vi "Begin.vi"(8 "error in":errorcluster) -> (0 "error out":errorcluster)   [LabVIEW 2017]
doc: "Called before other user functions, this VI is expected to open initial I/O refnums, load in file data, and do all program initialization. Notice that the <B>error out</B> terminal is simply used for data flow. Wiring it to other structures or subVIs ensures that this VI runs first."
uses:
  <vilib>/Rock Robotics/WPI/DriverStation/WPI_DriverStationRobotMode2.ctl
  <vilib>/Rock Robotics/WPI/Joystick/WPI_JoystickDeviceEnum.ctl
  <vilib>/Rock Robotics/WPI/Solenoid/WPI_SolenoidChannel.ctl
  <vilib>/Rock Robotics/SystemInterfaces/DIO/FPGA_DIOChannel.ctl
  <vilib>/Rock Robotics/SystemInterfaces/AI/FPGA_AIChannel.ctl
  Desktop/2018 FINAL/E/2018 FINAL/C/Users/admin/Documents/LabVIEW Data/2018 FINAL CODE/Robot Global Data.vi
  <vilib>/Rock Robotics/WPI/Solenoid/WPI_SolenoidOpenDouble.vi
  <vilib>/Rock Robotics/WPI/RobotDrive/WPI_RobotDriveOpen2MotorWithTalonSRX.vi
  <vilib>/Rock Robotics/WPI/ThirdParty/Phoenix-LabVIEW/Pigeon IMU/CTRE_PigeonIMU_Open_TalonSRX.vi
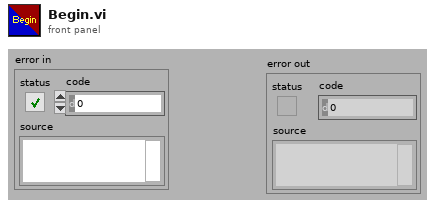
[diagram p1: front panel]
types:
  T1 = typedef "FPGA_AIChannel.ctl" = enum8{"AI 0", "AI 1", "AI 2", "AI 3", "AI MXP 0", "AI MXP 1", "AI MXP 2", "AI MXP 3", "Invalid"}
  T2 = typedef "FPGA_DIOChannel.ctl" = enum8{"DIO 0", "DIO 1", "DIO 2", "DIO 3", "DIO 4", "DIO 5", "DIO 6", "DIO 7", "DIO 8", "DIO 9", "DIO MXP 0", "DIO MXP 1", "DIO MXP 2", "DIO MXP 3", "DIO MXP 4", "DIO MXP 5", "DIO MXP 6", "DIO MXP 7", "DIO MXP 8", "DIO MXP 9", "DIO MXP 10", "DIO MXP 11", "DIO MXP 12", "DIO MXP 13", "DIO MXP 14", "DIO MXP 15", "SPI Port CS1", "SPI Port CS2", "SPI Port CS3", "SPI Port MISO", "SPI Port MOSI", "Invalid"}
  T3 = typedef "WPI_JoystickDeviceEnum.ctl" = enum16{"USB 0", "USB 1", "USB 2", "USB 3", "USB 4", "USB 5"}
  T4 = typedef "WPI_SolenoidChannel.ctl" = enum8{"Solenoid 0", "Solenoid 1", "Solenoid 2", "Solenoid 3", "Solenoid 4", "Solenoid 5", "Solenoid 6", "Solenoid 7", "Invalid"}
  T5 = typedef "WPI_DriverStationRobotMode2.ctl" = enum16{"Autonomous Disabled", "Autonomous Enabled", "Teleop Disabled", "Teleop Enabled", "Disconnected", "Finish", "Test Disabled", "Test Enabled", "Emergency Stopped"}
  T6 = typedef "WPI_MotorControlDeviceRef.ctl" = cluster{"DeviceStatus":errorcluster, "Type":T7, "PWM":cluster{"PWM Channel":T8, "DeadBand":T9}, "CAN":cluster{"Device Number":u8, "SetOutput VI Ref":variant, "GetOutput VI Ref":variant, "Enable VI Ref":variant, "Disable VI Ref":variant, "Data":variant}, "Invert":bool, "DIO PWM":cluster{"PWM \"Enable\" Channel":T8, "DIOChannel":T2, "PWM Rate":dbl}}
  T7 = typedef "WPI_MotorControlType.ctl" = enum16{"PWM", "CAN", "DIO PWM"}
  T8 = typedef "FPGA_DIOPWMChannel.ctl" = enum8{"PWM 0", "PWM 1", "PWM 2", "PWM 3", "PWM 4", "PWM 5", "PWM 6", "PWM 7", "PWM 8", "PWM 9", "PWM MXP 0", "PWM MXP 1", "PWM MXP 2", "PWM MXP 3", "PWM MXP 4", "PWM MXP 5", "PWM MXP 6", "PWM MXP 7", "PWM MXP 8", "PWM MXP 9", "Invalid"}
  T9 = typedef "WPI_PWMDeadband.ctl" = cluster{"Name":string, "maxPositivePwm":i32, "minPositivePwm":i32, "centerPwm":i32, "maxNegativePwm":i32, "minNegativePwm":i32, "angularRange":u16}
  T10 = typedef "WPI_JoystickDevRef.ctl" = cluster{"Device":T3}
  T11 = typedef "WPI_RobotDriveDevRef.ctl" = cluster{"DevStatus":errorcluster, "Motors[]":T6[], "Square Inputs":bool, "Max Output":dbl}
  T12 = typedef "WPI_SolenoidDevRef.ctl" = cluster{"DevStatus":errorcluster, "Pneumatics Control Module":u8, "Forward Solenoid Channel":T4, "Reverse Solenoid Channel":T4}
  T13 = typedef "CTRE_PigeonIMU_DeviceRef.ctl" = cluster{"DeviceStatus":errorcluster, "Device Number":u8, "Type":T14, "Device ID":u32, "Handle":u64, "UsageFrame":u32, "Library Path":path}
  T14 = typedef "CTRE_PigeonIMU_ConnectionType.ctl" = u32
  T15 = typedef "WPI_DigitalInputDevRef.ctl" = cluster{"DevStatus":errorcluster, "DIO Channel":T2}
  T16 = typedef "WPI_PotentiometerDevRef.ctl" = cluster{"DevStatus":errorcluster, "Analog Channel":T1, "Invert Output":bool}
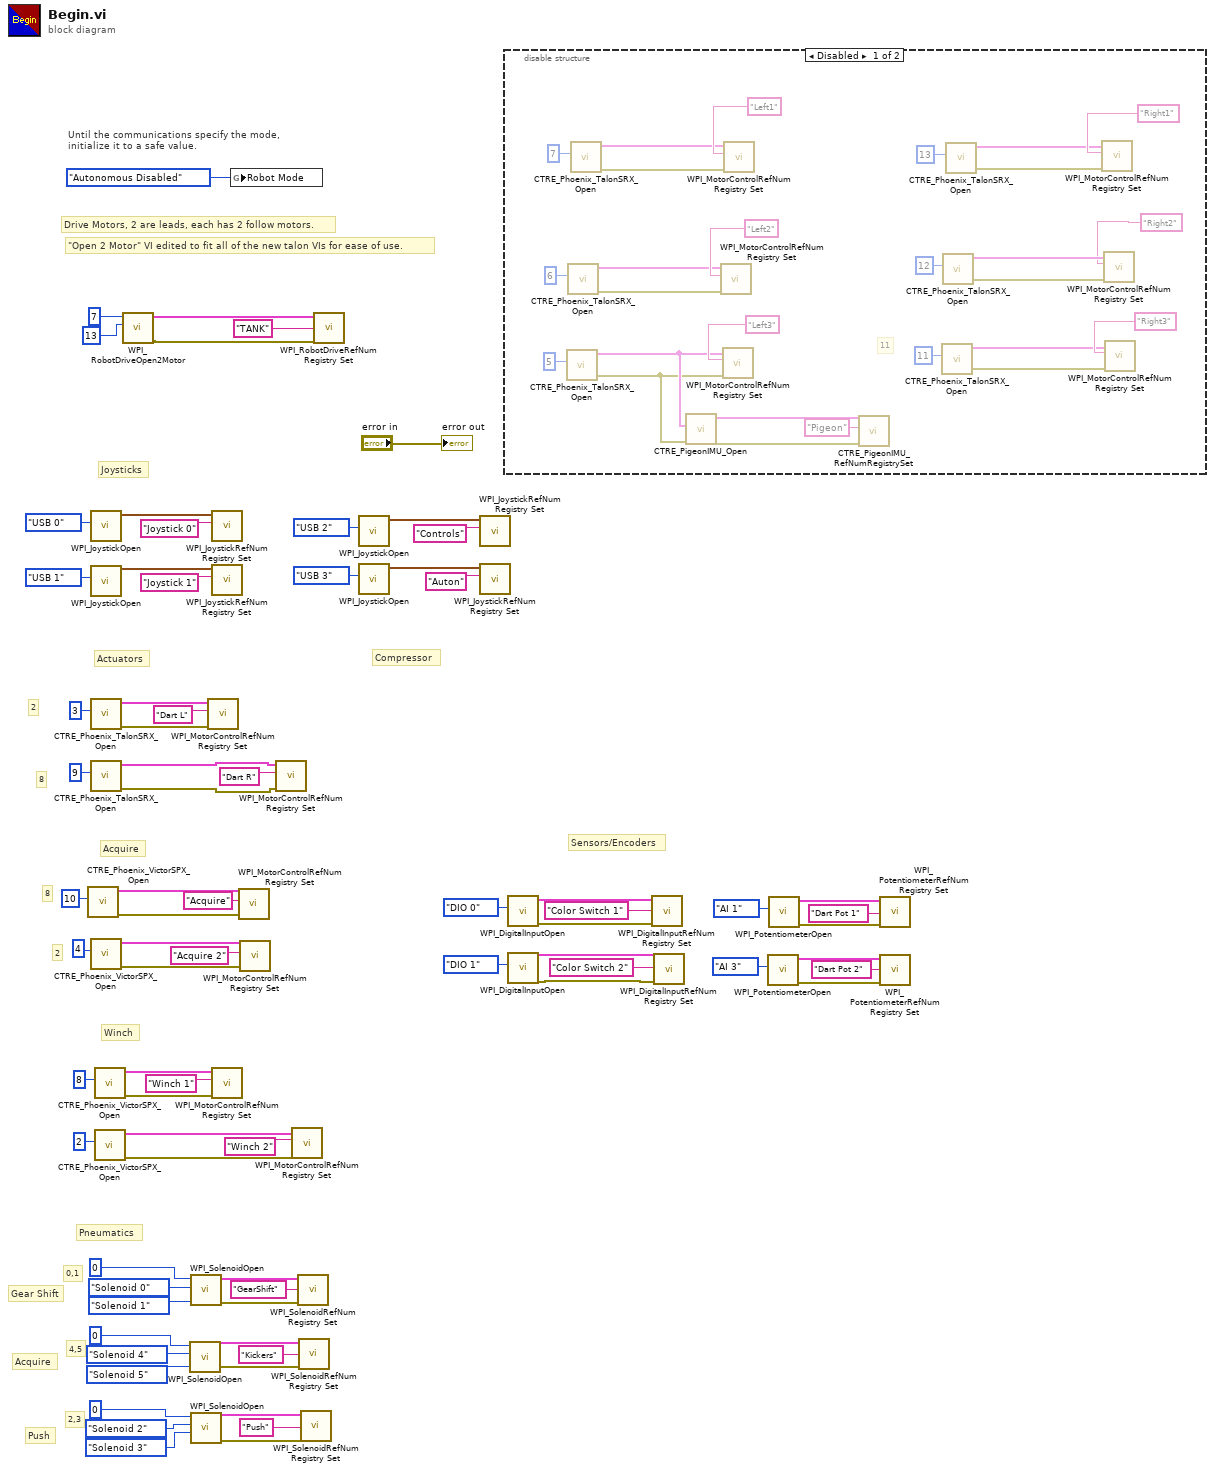
[diagram p0: block diagram]
diagram:
  # "2"
  # "8"
  # "2,3"
  # "4,5"
  # "0,1"
  # "Compressor"
  # "8"
  # "2"
  # "Winch"
  # "\"Open 2 Motor\" VI edited to fit all of the new talon VIs for ease of use."
  # "Sensors/Encoders"
  # "Acquire"
  # "Push"
  # "Acquire"
  # "Gear Shift"
  # "Pneumatics"
  # "Actuators"
  # "Joysticks"
  # "Drive Motors, 2 are leads, each has 2 follow motors."
  # "Until the communications specify the mode,\ninitialize it to a safe value."
  n1 = call <vilib>:"CTRE_Phoenix_VictorSPX_Open.vi"("Device Number"=u8 10) -> ("error out"=w7:errorcluster, "CAN Talon SRX Ref"=w8:T6)  [unwired: 9 in]
  n2 = call <vilib>:"WPI_JoystickOpen.vi"("JoystickDevice"=WPI_JoystickDeviceEnum."USB 0") -> ("JoystickDevRef"=w73:T10)  [unwired: 10 in]
  n3 = call <vilib>:"WPI_JoystickOpen.vi"("JoystickDevice"=WPI_JoystickDeviceEnum."USB 1") -> ("JoystickDevRef"=w70:T10)  [unwired: 10 in]
  n4 = call <vilib>:"CTRE_Phoenix_TalonSRX_Open.vi"("Device Number"=u8 3) -> ("error out"=w68:errorcluster, "CAN Talon SRX Ref"=w17:T6)  [unwired: 9 in]
  n5 = call <vilib>:"CTRE_Phoenix_TalonSRX_Open.vi"("Device Number"=u8 9) -> ("error out"=w15:errorcluster, "CAN Talon SRX Ref"=w16:T6)  [unwired: 9 in]
  n6 = call <vilib>:"CTRE_Phoenix_VictorSPX_Open.vi"("Device Number"=u8 4) -> ("error out"=w11:errorcluster, "CAN Talon SRX Ref"=w12:T6)  [unwired: 9 in]
  n7 = call <vilib>:"CTRE_Phoenix_VictorSPX_Open.vi"("Device Number"=u8 8) -> ("error out"=w24:errorcluster, "CAN Talon SRX Ref"=w21:T6)  [unwired: 9 in]
  n8 = call <vilib>:"CTRE_Phoenix_VictorSPX_Open.vi"("Device Number"=u8 2) -> ("error out"=w9:errorcluster, "CAN Talon SRX Ref"=w10:T6)  [unwired: 9 in]
  n9 = call-poly <vilib>:"WPI_RobotDriveOpen2Motor.vi"("Right"=u8 13 ("Right Lead"), "Left"=u8 7 ("Left Lead")) -> ("error out"=w3:errorcluster, "RobotDriveDevRef"=w4:T11)  [unwired: 8 in]
  n10 = call-poly <vilib>:"WPI_SolenoidOpen.vi"("Reverse Solenoid Channel"=WPI_SolenoidChannel."Solenoid 5", "Forward Solenoid Channel"=WPI_SolenoidChannel."Solenoid 4", "Pneumatics Control Module (0)"=u8 0) -> ("error out"=w55:errorcluster, "SolenoidDevRef"=w56:T12)  [unwired: 7 in]
  n11 = call-poly <vilib>:"WPI_SolenoidOpen.vi"("Reverse Solenoid Channel"=WPI_SolenoidChannel."Solenoid 1", "Forward Solenoid Channel"=WPI_SolenoidChannel."Solenoid 0", "Pneumatics Control Module (0)"=u8 0) -> ("error out"=w59:errorcluster, "SolenoidDevRef"=w58:T12)  [unwired: 7 in]
  n12 = call-poly <vilib>:"WPI_SolenoidOpen.vi"("Reverse Solenoid Channel"=WPI_SolenoidChannel."Solenoid 3", "Forward Solenoid Channel"=WPI_SolenoidChannel."Solenoid 2", "Pneumatics Control Module (0)"=u8 0) -> ("error out"=w52:errorcluster, "SolenoidDevRef"=w53:T12)  [unwired: 7 in]
  n13 = call <vilib>:"WPI_MotorControlRefNum Registry Set.vi"("error in (no error)"=w68, "refnum name"="Dart L", "MotorControlDevRef"=w17) -> ()  [unwired: 7 in, 2 out]
  n14 = call <vilib>:"WPI_JoystickRefNum Registry Set.vi"("refnum name"="Joystick 0", "JoystickDevRef"=w73) -> ()  [unwired: 8 in, 2 out]
  n15 = call <vilib>:"WPI_JoystickRefNum Registry Set.vi"("refnum name"="Joystick 1", "JoystickDevRef"=w70) -> ()  [unwired: 8 in, 2 out]
  n16 = call <vilib>:"WPI_MotorControlRefNum Registry Set.vi"("error in (no error)"=w24, "refnum name"="Winch 1", "MotorControlDevRef"=w21) -> ()  [unwired: 7 in, 2 out]
  n17 = global write "Robot Global Data.vi" "Robot Mode"(WPI_DriverStationRobotMode2."Autonomous Disabled" ("Robot Mode")) -> ()
  n18 = call <vilib>:"WPI_MotorControlRefNum Registry Set.vi"("error in (no error)"=w7, "refnum name"="Acquire", "MotorControlDevRef"=w8) -> ()  [unwired: 7 in, 2 out]
  n19 = call <vilib>:"WPI_MotorControlRefNum Registry Set.vi"("error in (no error)"=w11, "refnum name"="Acquire 2", "MotorControlDevRef"=w12) -> ()  [unwired: 7 in, 2 out]
  n20 = call <vilib>:"WPI_MotorControlRefNum Registry Set.vi"("error in (no error)"=w15, "refnum name"="Dart R", "MotorControlDevRef"=w16) -> ()  [unwired: 7 in, 2 out]
  n21 = call <vilib>:"WPI_MotorControlRefNum Registry Set.vi"("error in (no error)"=w9, "refnum name"="Winch 2", "MotorControlDevRef"=w10) -> ()  [unwired: 7 in, 2 out]
  n22 = call <vilib>:"WPI_SolenoidRefNum Registry Set.vi"("error in (no error)"=w59, "refnum name"="GearShift", "SolenoidDevRef"=w58) -> ()  [unwired: 7 in, 2 out]
  n23 = call <vilib>:"WPI_SolenoidRefNum Registry Set.vi"("error in (no error)"=w55, "refnum name"="Kickers", "SolenoidDevRef"=w56) -> ()  [unwired: 7 in, 2 out]
  n24 = call <vilib>:"WPI_SolenoidRefNum Registry Set.vi"("error in (no error)"=w52, "refnum name"="Push", "SolenoidDevRef"=w53) -> ()  [unwired: 7 in, 2 out]
  n25 = call <vilib>:"WPI_RobotDriveRefNum Registry Set.vi"("error in (no error)"=w3, "refnum name"="TANK", "RobotDriveDevRef"=w4) -> ()  [unwired: 7 in, 2 out]
  n26 = call <vilib>:"WPI_JoystickOpen.vi"("JoystickDevice"=WPI_JoystickDeviceEnum."USB 2") -> ("JoystickDevRef"=w49:T10)  [unwired: 10 in]
  n27 = call <vilib>:"WPI_JoystickOpen.vi"("JoystickDevice"=WPI_JoystickDeviceEnum."USB 3") -> ("JoystickDevRef"=w46:T10)  [unwired: 10 in]
  n28 = call <vilib>:"WPI_JoystickRefNum Registry Set.vi"("refnum name"="Controls", "JoystickDevRef"=w49) -> ()  [unwired: 8 in, 2 out]
  n29 = call <vilib>:"WPI_JoystickRefNum Registry Set.vi"("refnum name"="Auton", "JoystickDevRef"=w46) -> ()  [unwired: 8 in, 2 out]
  n30 = disable-structure shown="Disabled" {
    frame Disabled {
      # "11"
      n31 = call <vilib>:"CTRE_Phoenix_TalonSRX_Open.vi"("Device Number"=u8 5) -> ("error out"=w81:errorcluster, "CAN Talon SRX Ref"=w82:T6)  [unwired: 9 in]
      n32 = call <vilib>:"CTRE_Phoenix_TalonSRX_Open.vi"("Device Number"=u8 6) -> ("error out"=w96:errorcluster, "CAN Talon SRX Ref"=w97:T6)  [unwired: 9 in]
      n33 = call <vilib>:"CTRE_Phoenix_TalonSRX_Open.vi"("Device Number"=u8 7) -> ("error out"=w83:errorcluster, "CAN Talon SRX Ref"=w84:T6)  [unwired: 9 in]
      n34 = call-poly <vilib>:"CTRE_PigeonIMU_Open.vi"("error in"=w81, "CAN Talon SRX Ref"=w82) -> ("error out"=w79:errorcluster, "PigeonIMUDevRef"=w80:T13)  [unwired: 8 in]
      n35 = call <vilib>:"WPI_MotorControlRefNum Registry Set.vi"("error in (no error)"=w96, "refnum name"="Left2", "MotorControlDevRef"=w97) -> ()  [unwired: 7 in, 2 out]
      n36 = call <vilib>:"WPI_MotorControlRefNum Registry Set.vi"("error in (no error)"=w81, "refnum name"="Left3", "MotorControlDevRef"=w82) -> ()  [unwired: 7 in, 2 out]
      n37 = call <vilib>:"WPI_MotorControlRefNum Registry Set.vi"("error in (no error)"=w83, "refnum name"="Left1", "MotorControlDevRef"=w84) -> ()  [unwired: 7 in, 2 out]
      n38 = call <vilib>:"CTRE_PigeonIMU_RefNumRegistrySet.vi"("error in (no error)"=w79, "refnum name"="Pigeon", "PigeonIMUDevRef"=w80) -> ()  [unwired: 7 in, 2 out]
      n39 = call <vilib>:"CTRE_Phoenix_TalonSRX_Open.vi"("Device Number"=u8 11) -> ("error out"=w94:errorcluster, "CAN Talon SRX Ref"=w95:T6)  [unwired: 9 in]
      n40 = call <vilib>:"CTRE_Phoenix_TalonSRX_Open.vi"("Device Number"=u8 12) -> ("error out"=w92:errorcluster, "CAN Talon SRX Ref"=w93:T6)  [unwired: 9 in]
      n41 = call <vilib>:"CTRE_Phoenix_TalonSRX_Open.vi"("Device Number"=u8 13) -> ("error out"=w85:errorcluster, "CAN Talon SRX Ref"=w86:T6)  [unwired: 9 in]
      n42 = call <vilib>:"WPI_MotorControlRefNum Registry Set.vi"("error in (no error)"=w85, "refnum name"="Right1", "MotorControlDevRef"=w86) -> ()  [unwired: 7 in, 2 out]
      n43 = call <vilib>:"WPI_MotorControlRefNum Registry Set.vi"("error in (no error)"=w92, "refnum name"="Right2", "MotorControlDevRef"=w93) -> ()  [unwired: 7 in, 2 out]
      n44 = call <vilib>:"WPI_MotorControlRefNum Registry Set.vi"("error in (no error)"=w94, "refnum name"="Right3", "MotorControlDevRef"=w95) -> ()  [unwired: 7 in, 2 out]
    }
    frame Enabled {
    }
  }
  n45 = call <vilib>:"WPI_DigitalInputOpen.vi"("DIO Channel"=FPGA_DIOChannel."DIO 0") -> ("error out"=w40:errorcluster, "DigitalInputDevRef"=w41:T15)  [unwired: 9 in]
  n46 = call <vilib>:"WPI_DigitalInputOpen.vi"("DIO Channel"=FPGA_DIOChannel."DIO 1") -> ("error out"=w39:errorcluster, "DigitalInputDevRef"=w38:T15)  [unwired: 9 in]
  n47 = call <vilib>:"WPI_DigitalInputRefNum Registry Set.vi"("error in (no error)"=w40, "refnum name"="Color Switch 1", "DigitalInputDevRef"=w41) -> ()  [unwired: 7 in, 2 out]
  n48 = call <vilib>:"WPI_DigitalInputRefNum Registry Set.vi"("error in (no error)"=w39, "refnum name"="Color Switch 2", "DigitalInputDevRef"=w38) -> ()  [unwired: 7 in, 2 out]
  n49 = call <vilib>:"WPI_PotentiometerOpen.vi"("Analog Channel"=FPGA_AIChannel."AI 3") -> ("error out"=w29:errorcluster, "PotDevRef"=w28:T16)  [unwired: 9 in]
  n50 = call <vilib>:"WPI_PotentiometerOpen.vi"("Analog Channel"=FPGA_AIChannel."AI 1") -> ("error out"=w35:errorcluster, "PotDevRef"=w34:T16)  [unwired: 9 in]
  n51 = call <vilib>:"WPI_PotentiometerRefNum Registry Set.vi"("error in (no error)"=w35, "refnum name"="Dart Pot 1", "PotDevRef"=w34) -> ()  [unwired: 7 in, 2 out]
  n52 = call <vilib>:"WPI_PotentiometerRefNum Registry Set.vi"("error in (no error)"=w29, "refnum name"="Dart Pot 2", "PotDevRef"=w28) -> ()  [unwired: 7 in, 2 out]
  "error out" <- "error in"
